vi "Teleop.vi"(10 "Match Info":T1={"Autonomous Elapsed Seconds"=0.0, "TeleOp Elapsed Seconds"=0.0, "Disabled Elapsed Seconds"=0.0, "Visited Autonomous"=FALSE, "Visited TeleOp"=FALSE, "Visited Disabled"=FALSE, "Autonomous Settings"={"Autonomous Style"=enum."Independent", "VI Refnum"=refnum}}, 11 "Call Context":T2) -> ()   [LabVIEW 2016]
doc: "This VI is called for each TeleOp packet received from the DS where the robot is not disabled. It is often used to read from the joysticks and update I/O or to update setpoints for timed control loops. It should complete and return within 20 milliseconds or it may miss DS packets."
uses:
  <vilib>/Rock Robotics/WPI/DriverStation/WPI_DriverStationDerivedRobotMode.ctl
  <vilib>/Rock Robotics/WPI/DriverStation/WPI_DriverStationMatch Info.ctl
  <vilib>/Rock Robotics/WPI/Relay/WPI_RelayValue.ctl
  <vilib>/Rock Robotics/Network Tables/NT Read Number.vi
  <vilib>/Rock Robotics/Network Tables/NT Read Boolean.vi
  <vilib>/Rock Robotics/WPI/Utilities/WPI_GetSetVariantRefNum.vi
  <vilib>/Rock Robotics/Network Tables/NT Write Boolean Array.vi
  <vilib>/Rock Robotics/Network Tables/NT Write Numeric Array.vi
  <vilib>/Rock Robotics/WPI/Ultrasonic/WPI_SonarMB1010DigitalRefNum Registry Get.vi
  <vilib>/Rock Robotics/WPI/Ultrasonic/WPI_SonarMB1010DigitalGetRange.vi
  <vilib>/Rock Robotics/Network Tables/NT Write Number.vi
  <vilib>/gmath/NI_Gmath.lvlib
panel:
  out "Angle":dbl format="%#_13g"
  in  "Control Effort":dbl[](array[numeric])=[0.0, 0.0, 0.0, 0.0]
  in  "RPM Array":dbl[](array[numeric])=[0.0, 0.0, 0.0, 0.0]
  out "Encoder Index Count":dbl
  in  "OR Speed":dbl
  in  "Override?":bool
  out "Shooter RPM":dbl
  in  "kP":dbl=1.0 format="%#_13g"
  out "Shooter RPM":dbl(graph)
  in  "SET RPM":dbl format="%#_13g"
  in  "Tab Control":enum32{"Page 1", "Page 2"}(tab)
  out "Shooter Current":dbl
  out "Shooter Current":dbl(graph)
  out "Distance":dbl
  out "Sample Slider 0":dbl(slide) scale=0.0..5.0
  out "Sample Boolean 1":bool
  out "Sample Boolean 0":bool
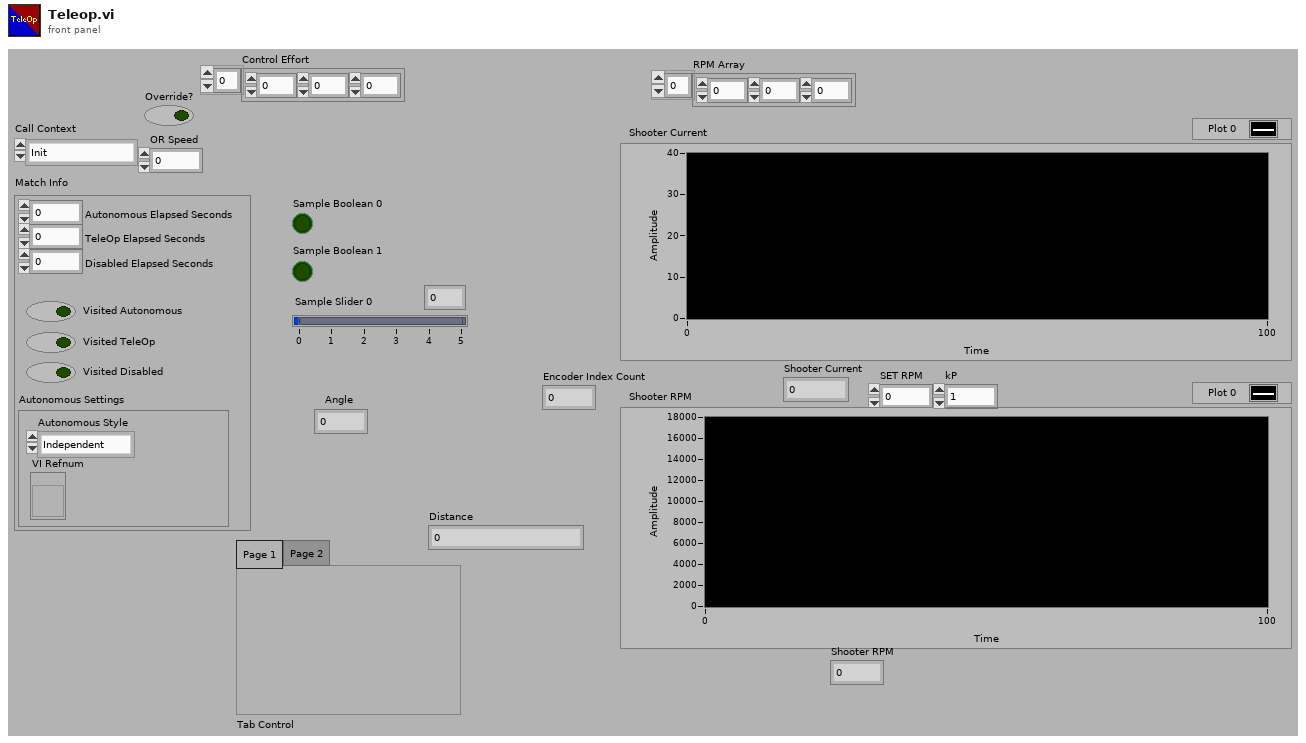
[diagram p1: front panel]
types:
  T1 = typedef "WPI_DriverStationMatch Info.ctl" = cluster{"Autonomous Elapsed Seconds":dbl, "TeleOp Elapsed Seconds":dbl, "Disabled Elapsed Seconds":dbl, "Visited Autonomous":bool, "Visited TeleOp":bool, "Visited Disabled":bool, "Autonomous Settings":cluster{"Autonomous Style":enum16{"Iterative", "Independent"}, "VI Refnum":refnum<vi>}}
  T2 = typedef "WPI_DriverStationDerivedRobotMode.ctl" = enum16{"Init", "Execute", "Stop"}
  T3 = typedef "WPI_MotorControlDeviceRef.ctl" = cluster{"DeviceStatus":errorcluster, "Type":T4, "PWM":cluster{"PWM Channel":T5, "DeadBand":T6}, "CAN":cluster{"Device Number":u8, "SetOutput VI Ref":variant, "GetOutput VI Ref":variant, "Enable VI Ref":variant, "Disable VI Ref":variant, "Data":variant}, "Invert":bool}
  T4 = typedef "WPI_MotorControlType.ctl" = enum16{"PWM", "CAN"}
  T5 = typedef "FPGA_DIOPWMChannel.ctl" = enum8{"PWM 0", "PWM 1", "PWM 2", "PWM 3", "PWM 4", "PWM 5", "PWM 6", "PWM 7", "PWM 8", "PWM 9", "PWM MXP 0", "PWM MXP 1", "PWM MXP 2", "PWM MXP 3", "PWM MXP 4", "PWM MXP 5", "PWM MXP 6", "PWM MXP 7", "PWM MXP 8", "PWM MXP 9", "Invalid"}
  T6 = typedef "WPI_PWMDeadband.ctl" = cluster{"Name":string, "maxPositivePwm":i32, "minPositivePwm":i32, "centerPwm":i32, "maxNegativePwm":i32, "minNegativePwm":i32, "angularRange":u16}
  T7 = typedef "WPI_CANTalonSRX_GlobalStatus.ctl" = cluster{"Applied Throttle":dbl, "Module Enabled":bool, "CAN Error":errorcluster, "Closed Loop Error":dbl, "Forward Limit Switch Closed":bool, "Reverse Limit Switch Closed":bool, "Sensor Position":dbl, "Sensor Velocity":dbl, "Current":dbl, "Sticky Fault - Over Temp":bool, "Sticky Fault - Under Voltage":bool, "Sticky Fault - Forward Limit":bool, "Sticky Fault - Reverse Limit":bool, "Sticky Fault - Forward Soft Limit":bool, "Sticky Fault - Reverse Soft Limit":bool, "Brake is Enabled":bool, "Encoder Position":dbl, "Encoder Velocity":dbl, "Encoder Index Count":dbl, "Encoder A Pin State":bool, "Encoder B Pin State":bool, "Encoder Index Pin State":bool, "Analog In":dbl, "Analog In Velocity":dbl, "Temperature (C)":dbl, "Battery Voltage":dbl, "Control 5 Is Supported":bool, "Current Profile Slot Select":dbl, "Pos Div 8":bool, "Vel Div 4":bool, "Pulse Width Position":i32, "Pulse Width Velocity":i32, "Pulse Width Rise To Rise (us)":i32, "Pulse Width Rise To Fall (us)":i32, "Mot Prof Active Is Under Run":bool, "Mot Prof Active Has Under Run":bool, "Mot Prof Active Is Last":bool, "Mot Prof Active Velocity Only":bool, "Mot Prof Active Is Valid":bool, "Mot Prof Buffer Is Full":bool, "Mot Prof Active Profile Slot Select":i32, "Mot Prof NextID":i32, "Mot Prof Count":i32, "Mot Prof Active Velocity":dbl, "Mot Prof Active Position":dbl, "Mot Prof Output Enable":i32}
  T8 = typedef "WPI_JoystickDevRef.ctl" = cluster{"Device":T9}
  T9 = typedef "WPI_JoystickDeviceEnum.ctl" = enum16{"USB 0", "USB 1", "USB 2", "USB 3", "USB 4", "USB 5"}
  T10 = typedef "WPI_SonarMB1010DigitalDeviceRef.ctl" = cluster{"CounterDevRef":T11, "Scaling factor (s/in)":dbl}
  T11 = typedef "WPI_CounterDevRef.ctl" = cluster{"DevStatus":errorcluster, "CntIndex":T12}
  T12 = typedef "FPGA_CounterCtrSystemIndex.ctl" = enum8{"Ctr 0", "Ctr 1", "Ctr 2", "Ctr 3", "Ctr 4", "Ctr 5", "Ctr 6", "Ctr 7", "Invalid"}
  T13 = typedef "WPI_GyroDevRef.ctl" = cluster{"DevStatus":errorcluster, "Analog Channel":T14, "Offset":dbl, "Gain (VoltsPerDegree/Second)":dbl, "Gyro Type":enum16{"Analog", "XRS450"}, "Handle":i32, "SPI Bus":T15, "Device Found":bool, "Sample Rate":dbl, "Calibrate On Open":bool}
  T14 = typedef "FPGA_AIChannel.ctl" = enum8{"AI 0", "AI 1", "AI 2", "AI 3", "AI MXP 0", "AI MXP 1", "AI MXP 2", "AI MXP 3", "Invalid"}
  T15 = typedef "spi_bus.ctl" = enum16{"SPI On-Board, CS0", "SPI On-Board, CS1", "SPI On-Board, CS2", "SPI On-Board, CS3", "SPI MXP", "Invalid"}
  T16 = typedef "WPI_RelayValue.ctl" = enum16{"Off", "On", "Forward", "Reverse"}
  T17 = typedef "WPI_RelayDevRef.ctl" = cluster{"DevStatus":errorcluster, "Relay Channel":T18, "Relay Direction":T19}
  T18 = typedef "FPGA_DIORelayChannel.ctl" = enum8{"Relay 0", "Relay 1", "Relay 2", "Relay 3", "Invalid"}
  T19 = typedef "WPI_RelayDirection.ctl" = enum16{"Both directions", "Forward only", "Reverse only"}
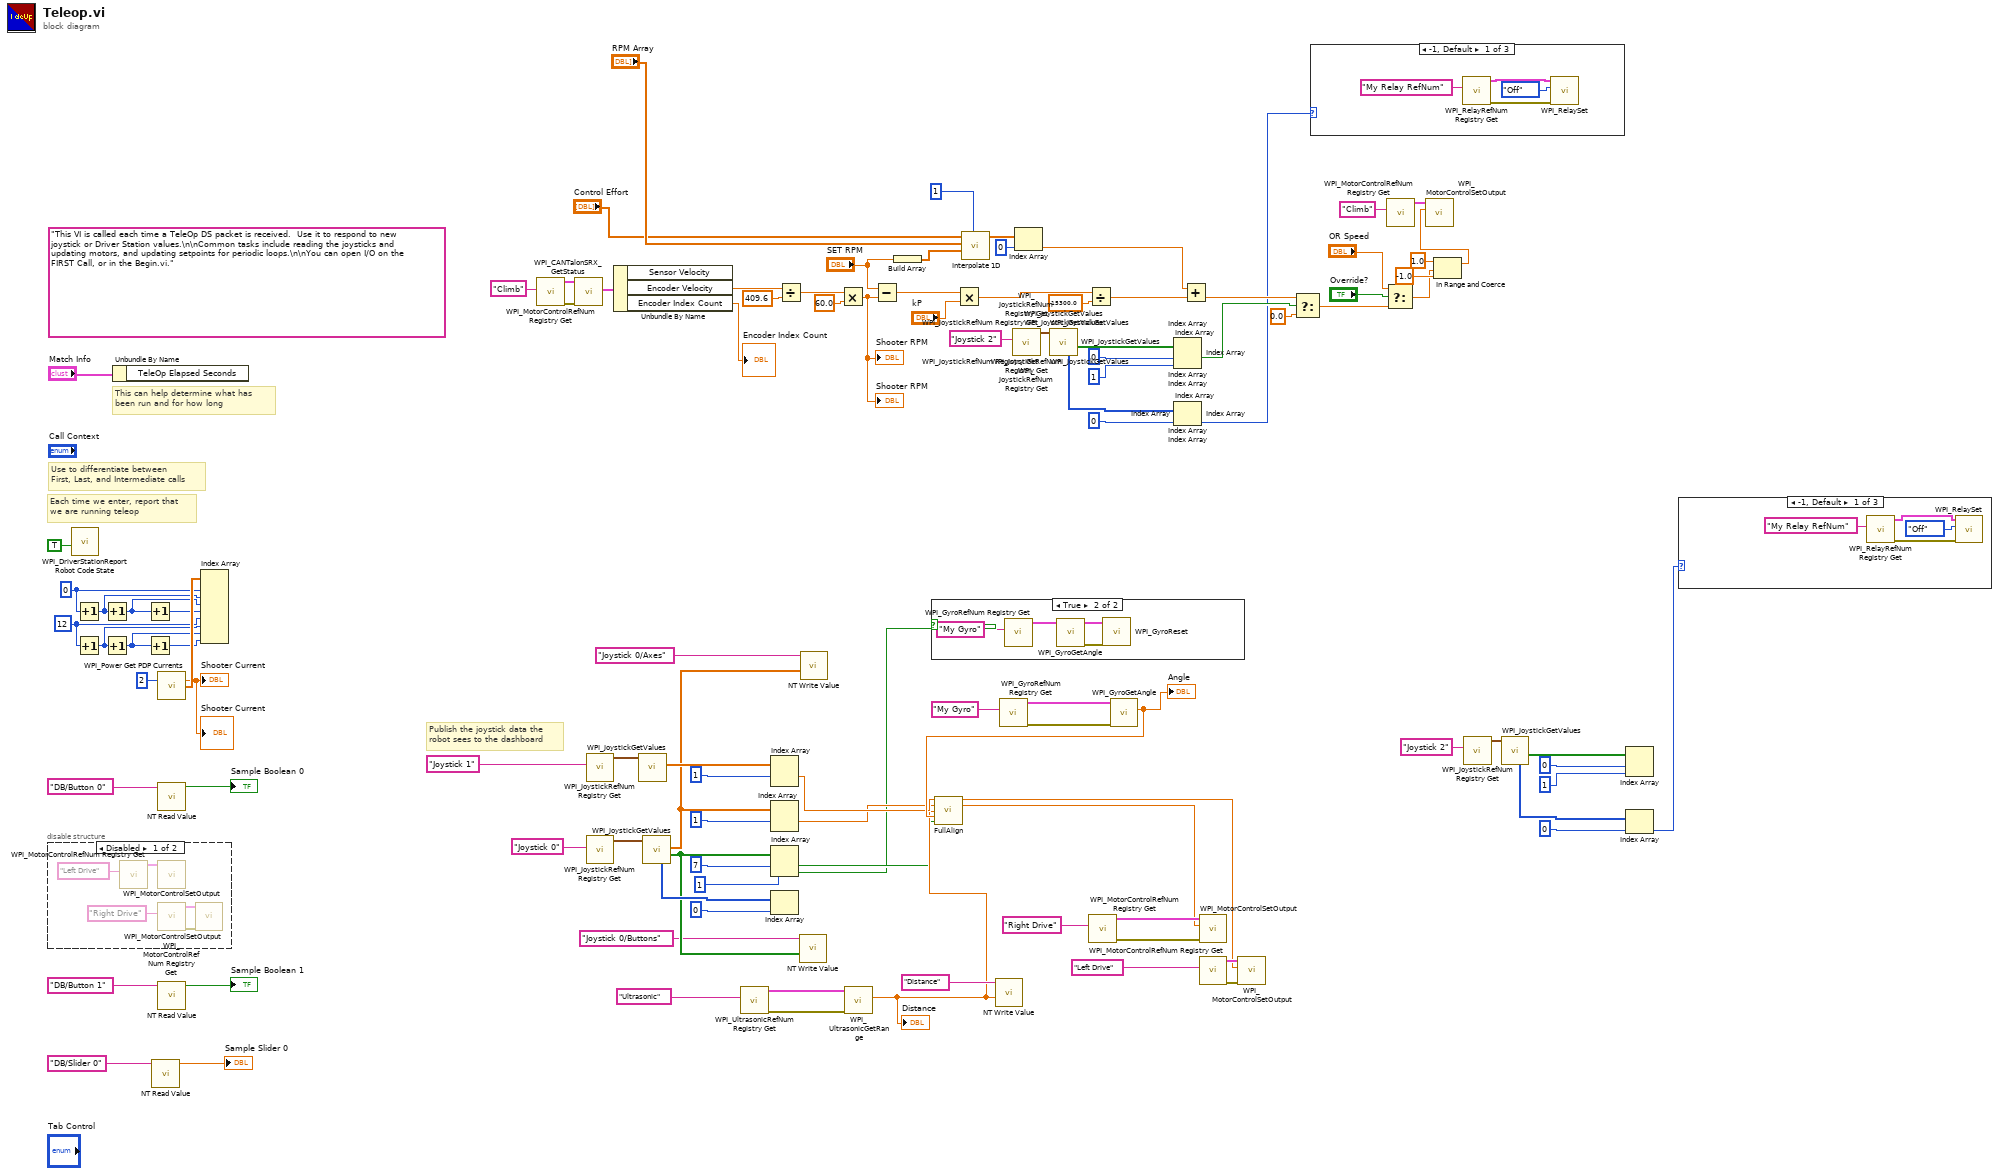
[diagram p0: block diagram]
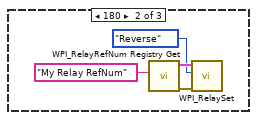
[diagram p2: hidden frame]
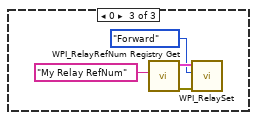
[diagram p3: hidden frame]
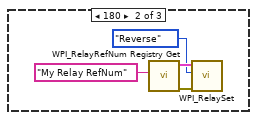
[diagram p4: hidden frame]
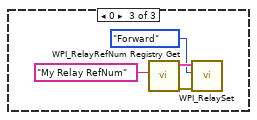
[diagram p5: hidden frame]
diagram:
  w125 = 12 ("PDP Channel")
  w129 = 0 ("PDP Channel")
  (unwired) "This VI is called each time a TeleOp DS packet is received.  Use it to respond to new joystick or Driver Station values.\n\nCommon tasks include reading the joysticks and updating motors, and updating setpoints for periodic loops.\n\nYou can open I/O on the FIRST Call, or in the Begin.vi."
  # "Publish the joystick data the\nrobot sees to the dashboard"
  # "Each time we enter, report that\nwe are running teleop"
  # "Use to differentiate between\nFirst, Last, and Intermediate calls"
  # "This can help determine what has\nbeen run and for how long"
  n1 = disable-structure shown="Disabled" {
    frame Disabled {
      n2 = call <vilib>:"WPI_MotorControlRefNum Registry Get.vi"("refnum name"="Left Drive") -> ("MotorControlDevRef"=w136:T3)  [unwired: 9 in, 1 out]
      n3 = call <vilib>:"WPI_MotorControlSetOutput.vi"("MotorControlDevRef"=w136) -> ()  [unwired: 8 in, 3 out]
      n4 = call <vilib>:"WPI_MotorControlRefNum Registry Get.vi"("refnum name"="Right Drive") -> ("error out"=w139:errorcluster, "MotorControlDevRef"=w138:T3)  [unwired: 9 in]
      n5 = call <vilib>:"WPI_MotorControlSetOutput.vi"("error in (no error)"=w139, "MotorControlDevRef"=w138) -> ()  [unwired: 7 in, 3 out]
    }
    frame Enabled {
    }
  }
  n6 = call <vilib>:"WPI_DriverStationReport Robot Code State.vi"("TeleOp"=TRUE ("Autonomous")) -> ()  [unwired: 10 in, 1 out]
  n7 = Increment(x=w129) -> (x+1=w128:i32)
  n8 = Increment(x=w125) -> (x+1=w124:i32)
  n9 = Increment(x=w128) -> (x+1=w126:i32)
  n10 = Increment(x=w124) -> (x+1=w122:i32)
  n11 = Unbundle By Name("Match Info") -> ()  [unwired: 1 out]
  n12 = Increment(x=w126) -> (x+1=w127:i32)
  n13 = Increment(x=w122) -> (x+1=w123:i32)
  n14 = call-poly <vilib>:"NT Read Value.vi"("Name"="DB/Slider 0" ("refnum name")) -> ("Numeric"=→"Sample Slider 0":dbl)  [unwired: 9 in, 1 out]
  n15 = call <vilib>:"WPI_Power Get PDP Currents.vi"("PDP Channel"=2) -> ("current (A)"=→"Shooter Current" →"Shooter Current":dbl, "all currents (A)"=w130:dbl[])  [unwired: 12 in, 1 out]
  n16 = call-poly <vilib>:"NT Read Value.vi"("Name"="DB/Button 0" ("refnum name")) -> ("Boolean"=→"Sample Boolean 0":bool)  [unwired: 9 in, 1 out]
  n17 = call-poly <vilib>:"NT Read Value.vi"("Name"="DB/Button 1" ("refnum name")) -> ("Boolean"=→"Sample Boolean 1":bool)  [unwired: 9 in, 1 out]
  n18 = Index Array(array=w130, index #1=w129, index #2=w128, index #3=w126, index #4=w127, index #5=w125, index #6=w124, index #7=w122, index #8=w123) -> ()  [unwired: 8 out]
  n19 = call <vilib>:"WPI_MotorControlRefNum Registry Get.vi"("refnum name"="Climb") -> ("error out"=w21:errorcluster, "MotorControlDevRef"=w20:T3)  [unwired: 9 in]
  n20 = call <vilib>:"WPI_CANTalonSRX_GetStatus.vi"("error in (no error)"=w21, "CAN Talon SRX Ref"=w20) -> ("Talon SRX Status"=w30:T7)  [unwired: 7 in, 2 out]
  n21 = call <vilib>:"WPI_JoystickRefNum Registry Get.vi"("refnum name"="Joystick 1") -> ("JoystickDevRef"=w95:T8)  [unwired: 1 in, 9 out]
  n22 = call <vilib>:"WPI_JoystickRefNum Registry Get.vi"("refnum name"="Joystick 0") -> ("JoystickDevRef"=w90:T8)  [unwired: 1 in, 9 out]
  n23 = Unbundle By Name(w30) -> ("Encoder Velocity"=w24:dbl, "Encoder Index Count"=→"Encoder Index Count":dbl)  [unwired: 1 out]
  n24 = call <vilib>:"WPI_JoystickGetValues.vi"("JoystickDevRef"=w95) -> ("Axes"=w94:dbl[])  [unwired: 6 in, 4 out]
  n25 = call <vilib>:"WPI_JoystickGetValues.vi"("JoystickDevRef"=w90) -> ("Buttons"=w103:bool[], "Axes"=w93:dbl[], "POVs"=w114:i16[])  [unwired: 6 in, 2 out]
  n26 = call-poly <vilib>:"WPI_UltrasonicRefNum Registry Get.vi"("refnum name"="Ultrasonic") -> ("error out"=w100:errorcluster, "SonarMB1010DigitalDevRef"=w101:T10)  [unwired: 9 in]
  n27 = Index Array(array=w94, index #1=1 ("index")) -> (element #1=w79:dbl)  [unwired: 1 in, 1 out]
  n28 = Index Array(array=w93, index #1=1 ("index")) -> (element #1=w78:dbl)  [unwired: 1 in, 1 out]
  n29 = Index Array(array=w103, index #1=7 ("index"), index #2=1) -> (element #1=w76:bool, element #2=w72:bool)
  n30 = Index Array(array=w114, index=0) -> ()  [unwired: 1 out]
  n31 = Divide(x=w24, y=409.6) -> (x/y=w23:dbl)
  n32 = call-poly <vilib>:"NT Write Value.vi"("Boolean Array"=w103, "Name"="Joystick 0/Buttons") -> ()  [unwired: 9 in, 1 out]
  n33 = call-poly <vilib>:"NT Write Value.vi"("Numeric Array"=w93, "Name"="Joystick 0/Axes") -> ()  [unwired: 9 in, 1 out]
  n34 = Multiply(x=w23, y=60.0) -> (x*y=w26:dbl)
  "Shooter RPM" <- w26
  "Shooter RPM" <- w26
  n35 = call-poly <vilib>:"WPI_UltrasonicGetRange.vi"("error in"=w100, "SonarMB1010DigitalDevRef"=w101) -> ("Distance"=w77:dbl)  [unwired: 7 in, 2 out]
  "Distance" <- w77
  n36 = Subtract(x="SET RPM", y=w26) -> (x-y=w11:dbl)
  n37 = Build Array("SET RPM") -> (w35:dbl[])
  n38 = case shown="True" w72 {
    frame False {
    }
    frame True {
      n39 = call <vilib>:"WPI_GyroRefNum Registry Get.vi"("refnum name"="My Gyro") -> ("GyroDevRef"=w142:T13)  [unwired: 9 in, 1 out]
      n40 = call <vilib>:"WPI_GyroGetAngle.vi"("GyroDevRef"=w142) -> ("error out"=w141:errorcluster, "GyroDevRef"=w140:T13)  [unwired: 6 in, 3 out]
      n41 = call <vilib>:"WPI_GyroReset.vi"("error in"=w141, "GyroDevRef"=w140) -> ()  [unwired: 8 in, 2 out]
    }
  }
  n42 = Multiply(x=w11, y="kP") -> (x*y=w29:dbl)
  n43 = call <vilib>:"Interpolate 1D.vi"("method"=1, "xi"=w35, "X"="RPM Array", "Y"="Control Effort") -> ("yi"=w36:dbl[])  [unwired: 5 in, 2 out]
  n44 = call-poly <vilib>:"NT Write Value.vi"("Numeric"=w77, "Name"="Distance") -> ()  [unwired: 9 in, 1 out]
  n45 = call <vilib>:"WPI_GyroRefNum Registry Get.vi"("refnum name"="My Gyro") -> ("error out"=w113:errorcluster, "GyroDevRef"=w112:T13)  [unwired: 9 in]
  n46 = call <vilib>:"WPI_JoystickRefNum Registry Get.vi"("refnum name"="Joystick 2") -> ("JoystickDevRef"=w70:T8)  [unwired: 1 in, 9 out]
  n47 = call <vilib>:"WPI_JoystickRefNum Registry Get.vi"("refnum name"="Joystick 2") -> ("JoystickDevRef"=w63:T8)  [unwired: 1 in, 9 out]
  n48 = call <vilib>:"WPI_JoystickRefNum Registry Get.vi"("refnum name"="Joystick 2") -> ("JoystickDevRef"=w52:T8)  [unwired: 1 in, 9 out]
  n49 = call <vilib>:"WPI_JoystickRefNum Registry Get.vi"("refnum name"="Joystick 2") -> ("JoystickDevRef"=w49:T8)  [unwired: 1 in, 9 out]
  n50 = call <vilib>:"WPI_JoystickRefNum Registry Get.vi"("refnum name"="Joystick 2") -> ("JoystickDevRef"=w6:T8)  [unwired: 1 in, 9 out]
  n51 = Index Array(array=w36, index=0) -> (element=w39:dbl)
  n52 = call <vilib>:"WPI_JoystickGetValues.vi"("JoystickDevRef"=w70) -> ("Buttons"=w68:bool[], "POVs"=w65:i16[])  [unwired: 6 in, 3 out]
  n53 = call <vilib>:"WPI_JoystickGetValues.vi"("JoystickDevRef"=w63) -> ("Buttons"=w61:bool[], "POVs"=w58:i16[])  [unwired: 6 in, 3 out]
  n54 = call <vilib>:"WPI_JoystickGetValues.vi"("JoystickDevRef"=w52) -> ("Buttons"=w54:bool[], "POVs"=w57:i16[])  [unwired: 6 in, 3 out]
  n55 = call <vilib>:"WPI_JoystickGetValues.vi"("JoystickDevRef"=w49) -> ("Buttons"=w47:bool[], "POVs"=w44:i16[])  [unwired: 6 in, 3 out]
  n56 = call <vilib>:"WPI_JoystickGetValues.vi"("JoystickDevRef"=w6) -> ("Buttons"=w8:bool[], "POVs"=w14:i16[])  [unwired: 6 in, 3 out]
  n57 = Divide(x=w29, y=15300.0) -> (x/y=w28:dbl)
  n58 = call <vilib>:"WPI_MotorControlRefNum Registry Get.vi"("refnum name"="Right Drive") -> ("error out"=w105:errorcluster, "MotorControlDevRef"=w106:T3)  [unwired: 9 in]
  n59 = call <vilib>:"WPI_GyroGetAngle.vi"("error in"=w113, "GyroDevRef"=w112) -> ("Angle"=w80:dbl)  [unwired: 5 in, 4 out]
  "Angle" <- w80
  n60 = call "FullAlign.vi"("Joystick 0"=w79, "Joystick 1"=w78, "Distance"=w77, "Angle"=w80, "Button"=w76) -> ("Right Motor"=w75:dbl, "Left Motor"=w74:dbl)  [unwired: 6 in, 3 out]
  n61 = Index Array(array=w68, index #1=0 ("index"), index #2=1 ("index")) -> (element #1=w2:bool)  [unwired: 1 out]
  n62 = Index Array(array=w61, index #1=0 ("index"), index #2=1 ("index")) -> ()  [unwired: 2 out]
  n63 = Index Array(array=w54, index #1=0 ("index"), index #2=1 ("index")) -> ()  [unwired: 2 out]
  n64 = Index Array(array=w47, index #1=0 ("index"), index #2=1 ("index")) -> ()  [unwired: 2 out]
  n65 = Index Array(array=w8, index #1=0 ("index"), index #2=1 ("index")) -> ()  [unwired: 2 out]
  n66 = Index Array(array=w65, index=0) -> (element=w1:i16)
  n67 = Index Array(array=w58, index=0) -> ()  [unwired: 1 out]
  n68 = Index Array(array=w57, index=0) -> ()  [unwired: 1 out]
  n69 = Index Array(array=w44, index=0) -> ()  [unwired: 1 out]
  n70 = Index Array(array=w14, index=0) -> ()  [unwired: 1 out]
  n71 = Add(x=w39, y=w28) -> (x+y=w38:dbl)
  n72 = call <vilib>:"WPI_MotorControlSetOutput.vi"("error in (no error)"=w105, "Output"=w74, "MotorControlDevRef"=w106) -> ()  [unwired: 6 in, 3 out]
  n73 = call <vilib>:"WPI_MotorControlRefNum Registry Get.vi"("refnum name"="Left Drive") -> ("error out"=w110:errorcluster, "MotorControlDevRef"=w109:T3)  [unwired: 9 in]
  n74 = call <vilib>:"WPI_MotorControlSetOutput.vi"("error in (no error)"=w110, "Output"=w75, "MotorControlDevRef"=w109) -> ()  [unwired: 6 in, 3 out]
  n75 = Select(t=w38, s=w2, f=0.0) -> (s? t:f=w18:dbl)
  n76 = case shown="-1, Default" w1 {
    frame -1, Default {
      n77 = call <vilib>:"WPI_RelayRefNum Registry Get.vi"("refnum name"="My Relay RefNum") -> ("error out"=w147:errorcluster, "RelayDevRef"=w146:T17)  [unwired: 9 in]
      n78 = call <vilib>:"WPI_RelaySet.vi"("error in (no error)"=w147, "RelayValue"=WPI_RelayValue."Off", "RelayDevRef"=w146) -> ()  [unwired: 7 in, 2 out]
    }
    frame 180 {
      n79 = call <vilib>:"WPI_RelayRefNum Registry Get.vi"("refnum name"="My Relay RefNum") -> ("error out"=w151:errorcluster, "RelayDevRef"=w150:T17)  [unwired: 9 in]
      n80 = call <vilib>:"WPI_RelaySet.vi"("error in (no error)"=w151, "RelayValue"=WPI_RelayValue."Reverse", "RelayDevRef"=w150) -> ()  [unwired: 7 in, 2 out]
    }
    frame 0 {
      n81 = call <vilib>:"WPI_RelayRefNum Registry Get.vi"("refnum name"="My Relay RefNum") -> ("error out"=w155:errorcluster, "RelayDevRef"=w154:T17)  [unwired: 9 in]
      n82 = call <vilib>:"WPI_RelaySet.vi"("error in (no error)"=w155, "RelayValue"=WPI_RelayValue."Forward", "RelayDevRef"=w154) -> ()  [unwired: 7 in, 2 out]
    }
  }
  n83 = Select(t="OR Speed", s="Override?", f=w18) -> (s? t:f=w40:dbl)
  n84 = call <vilib>:"WPI_MotorControlRefNum Registry Get.vi"("refnum name"="Climb") -> ("MotorControlDevRef"=w3:T3)  [unwired: 9 in, 1 out]
  n85 = In Range and Coerce(upper limit=1.0, x=w40, lower limit=-1.0) -> (coerced(x)=w43:dbl)  [unwired: 1 out]
  n86 = call <vilib>:"WPI_MotorControlSetOutput.vi"("Output"=w43, "MotorControlDevRef"=w3) -> ()  [unwired: 7 in, 3 out]
  n87 = call <vilib>:"WPI_JoystickRefNum Registry Get.vi"("refnum name"="Joystick 2") -> ("JoystickDevRef"=w83:T8)  [unwired: 1 in, 9 out]
  n88 = call <vilib>:"WPI_JoystickGetValues.vi"("JoystickDevRef"=w83) -> ("Buttons"=w85:bool[], "POVs"=w88:i16[])  [unwired: 6 in, 3 out]
  n89 = Index Array(array=w85, index #1=0 ("index"), index #2=1 ("index")) -> ()  [unwired: 2 out]
  n90 = Index Array(array=w88, index=0) -> (element=w81:i16)
  n91 = case shown="-1, Default" w81 {
    frame -1, Default {
      n92 = call <vilib>:"WPI_RelayRefNum Registry Get.vi"("refnum name"="My Relay RefNum") -> ("error out"=w159:errorcluster, "RelayDevRef"=w158:T17)  [unwired: 9 in]
      n93 = call <vilib>:"WPI_RelaySet.vi"("error in (no error)"=w159, "RelayValue"=WPI_RelayValue."Off", "RelayDevRef"=w158) -> ()  [unwired: 7 in, 2 out]
    }
    frame 180 {
      n94 = call <vilib>:"WPI_RelayRefNum Registry Get.vi"("refnum name"="My Relay RefNum") -> ("error out"=w163:errorcluster, "RelayDevRef"=w162:T17)  [unwired: 9 in]
      n95 = call <vilib>:"WPI_RelaySet.vi"("error in (no error)"=w163, "RelayValue"=WPI_RelayValue."Reverse", "RelayDevRef"=w162) -> ()  [unwired: 7 in, 2 out]
    }
    frame 0 {
      n96 = call <vilib>:"WPI_RelayRefNum Registry Get.vi"("refnum name"="My Relay RefNum") -> ("error out"=w167:errorcluster, "RelayDevRef"=w166:T17)  [unwired: 9 in]
      n97 = call <vilib>:"WPI_RelaySet.vi"("error in (no error)"=w167, "RelayValue"=WPI_RelayValue."Forward", "RelayDevRef"=w166) -> ()  [unwired: 7 in, 2 out]
    }
  }
